vi "设置转动方向.vi"(8 "error in (no error)":errorcluster caption="错误输入（无错误）", 10 "方向":bool, 11 "Hardware Resources in":T1 caption="硬件资源输入") -> (0 "error out":errorcluster caption="错误输出", 3 "Hardware Resources out":T1 caption="硬件资源输出")   [LabVIEW 2015, in "Action.lvlib"]
doc: "初始化硬件引用。"
uses:
  Action.lvlib
  <vilib>/DAQmx/write.llb/DAQmx Write (Digital Bool 1Line 1Point).vi
  <vilib>/DAQmx/create/channels.llb/DAQmx Create Channel (DO-Digital Output).vi
  <vilib>/DAQmx/miscellaneous.llb/DAQmx Fill In Error Info.vi
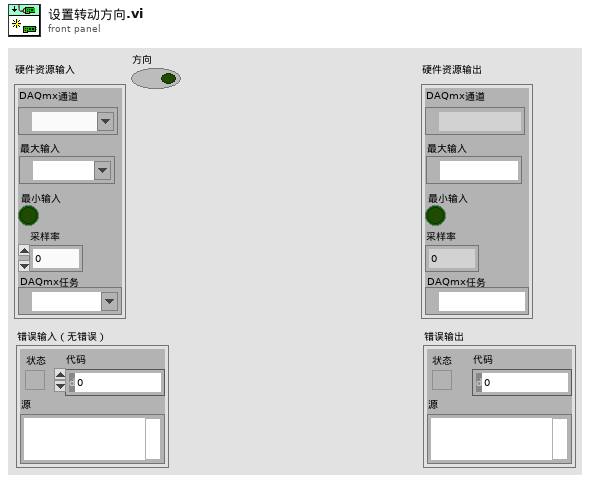
[diagram p1: front panel]
types:
  T1 = typedef "Action.lvlib/电机控制设置.ctl" = cluster{"counter":tag, "方向端口":tag, "当前方向":bool, "频率":dbl, "DAQmx Task":refnum<k21>}
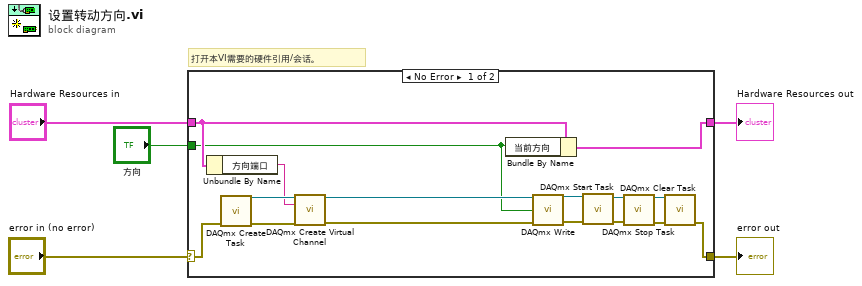
[diagram p0: block diagram]
diagram:
  # "打开本VI需要的硬件引用/会话。"
  n1 = case shown="No Error" "error in (no error)" {
    selector: "error in (no error)" -> [w13 w22]
    tunnel: [w12 w22] -> w4
    tunnel: "Hardware Resources in" -> [w10 w23]
    tunnel: [w8 w23] -> w2
    tunnel: "方向" -> [w6 _]
    frame No Error {
      n2 = Unbundle By Name(w10) -> ("方向端口"=w11:tag)
      n3 = call <vilib>:"DAQmx Create Task.vi"("error in"=w13) -> ("task out"=w20:refnum<k21>, "error out"=w21:errorcluster)  [unwired: 13 in]
      n4 = call-poly <vilib>:"DAQmx Create Virtual Channel.vi"("task in"=w20, "lines"=w11, "error in"=w21) -> ("task out"=w9:refnum<k21>, "error out"=w14:errorcluster)  [unwired: 11 in]
      n5 = Bundle By Name(cluster=w10, "当前方向"=w6) -> (w8:T1)
      n6 = call-poly <vilib>:"DAQmx Write.vi"("task/channels in"=w9, "data"=w6, "error in"=w14) -> ("task out"=w7:refnum<k21>, "error out"=w19:errorcluster)  [unwired: 10 in, 1 out]
      n7 = call <vilib>:"DAQmx Start Task.vi"("task/channels in"=w7, "error in"=w19) -> ("task out"=w17:refnum<k21>, "error out"=w18:errorcluster)  [unwired: 12 in]
      n8 = call <vilib>:"DAQmx Stop Task.vi"("task/channels in"=w17, "error in"=w18) -> ("task out"=w15:refnum<k21>, "error out"=w16:errorcluster)  [unwired: 12 in]
      n9 = call <vilib>:"DAQmx Clear Task.vi"("task in"=w15, "error in"=w16) -> ("error out"=w12:errorcluster)  [unwired: 13 in]
    }
    frame Error {
    }
  }
  "Hardware Resources out" <- w2
  "error out" <- w4
